vi "getFiducial.vi"(8 "error in (no error)":errorcluster, 9 "interactive":i32, 10 "Fiducial Parameters":T2, 11 "Image Parameters":T1) -> (0 "error out":errorcluster, 1 "coords":sgl[](array[numeric]), 2 "numFiducials":i32)   [LabVIEW 2011, in "gVision.lvlib"]
uses:
  gVision.lvlib
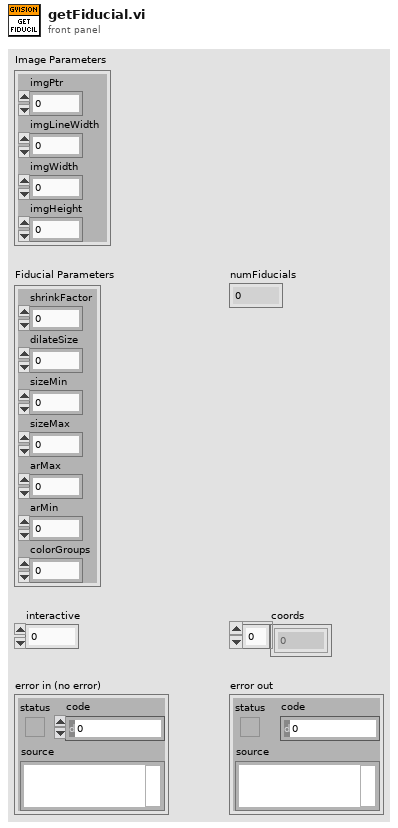
[diagram p1: front panel]
types:
  T1 = cluster{"imgPtr":i32, "imgLineWidth":i32, "imgWidth":i32, "imgHeight":i32}
  T2 = cluster{"shrinkFactor":sgl, "dilateSize":i32, "sizeMin":sgl, "sizeMax":sgl, "arMin":sgl, "arMax":sgl, "colorGroups":i32}
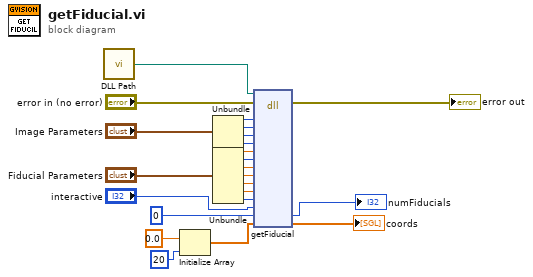
[diagram p0: block diagram]
diagram:
  n1 = call "DLL Path.vi"() -> ("DLL Path"=w1:path)  [unwired: 5 in]
  n2 = Initialize Array(0.0 ("element"), 20 ("dimension size")) -> (w19:dbl[])
  n3 = Unbundle("Image Parameters") -> ("imgPtr"=w7:i32, "imgLineWidth"=w6:i32, "imgWidth"=w5:i32, "imgHeight"=w4:i32)
  n4 = Unbundle("Fiducial Parameters") -> ("shrinkFactor"=w15:sgl, "dilateSize"=w9:i32, "sizeMin"=w10:sgl, "sizeMax"=w11:sgl, "arMin"=w12:sgl, "arMax"=w13:sgl, "colorGroups"=w14:i32)
  n5 = dll-call lib="?" fn="getFiducial"(path in=w1, error in="error in (no error)", "imgPtr"=w7, "imgLineWidth"=w6, "imgWidth"=w5, "imgHeight"=w4, "shrinkFactor"=w15, "dilateSize"=w9, "sizeMin"=w10, "sizeMax"=w11, "arMin"=w12, "arMax"=w13, "colorGroups"=w14, "interactive"="interactive", "numFiducials"=0, "coords"=w19) -> (error out=→"error out":errorcluster, "numFiducials"=→"numFiducials":i32, "coords"=→"coords":sgl[])  [unwired: 14 in, 1 out]
